vi "Assert Not Equal Value and Type_Variant.vi"(4 "Execution time (s)":dbl=-1.0, 6 "error code (1)":i32=1, 7 "Label":string, 8 "error in":errorcluster, 10 "Y":variant, 11 "X":variant) -> (0 "error out":errorcluster, 2 "Properties":refnum<class "Properties.Assert.lvclass">)   [LabVIEW 2021, in "Banana.Caraya.lvlib" / "Platano.CarayaTestSuite.lvclass"]
uses:
  Platano.CarayaTestSuite.lvclass
  Platano.CarayaTestSuite.lvclass/Platano.CarayaTestSuite.ctl
  <vilib>/addons/_JKI Toolkits/Caraya/classes/Assert/Assert.lvclass
  Bananas/Platano/Platano.lvclass
  Bananas/Banana/Banana.lvclass
  Bananas/AssertEqualType/AssertEqualType.lvclass
  Bananas/AssertEqualValue/AssertEqualValue.lvclass
  Properties.Banana/Properties.Banana.lvclass
  <vilib>/addons/_JKI Toolkits/Caraya/classes/Properties.Assert/Properties.Assert.lvclass
  C:/Program Files (x86)/National Instruments/LabVIEW 2021/vi.lib/addons/_JKI Toolkits/Caraya/classes/Properties/Properties.lvclass
  C:/Program Files (x86)/National Instruments/LabVIEW 2021/vi.lib/addons/_JKI Toolkits/Caraya/classes/Properties.Assert/Properties.Assert.lvclass
  C:/Repositories/LVOS/Bananas/lv-src/Bananas/AssertEqualValue/AssertEqualValue.lvclass
  C:/Repositories/LVOS/Bananas/lv-src/Bananas/BananaPeel/BananaPeel.lvclass
  C:/Repositories/LVOS/Bananas/lv-src/Bananas/AssertEqualType/AssertEqualType.lvclass
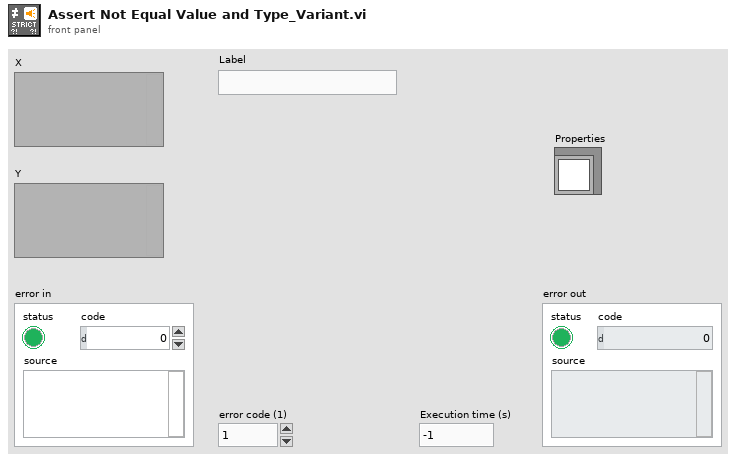
[diagram p1: front panel]
types:
  T1 = typedef "Bananas.lvlib/Assertion Strategies -- cluster.ctl" = cluster{"AssertTrue":refnum<class "AssertTrue.lvclass">, "AssertFalse":refnum<class "AssertFalse.lvclass">, "AssertEqualValue":refnum<class "AssertEqualValue.lvclass">, "AssertEqualType":refnum<class "AssertEqualType.lvclass">, "AssertCompareValue":refnum<class "AssertCompareValue.lvclass">, "AssertError":refnum<class "AssertError.lvclass">, "AssertAlmostEqual":refnum<class "AssertAlmostEqualValue.lvclass">}
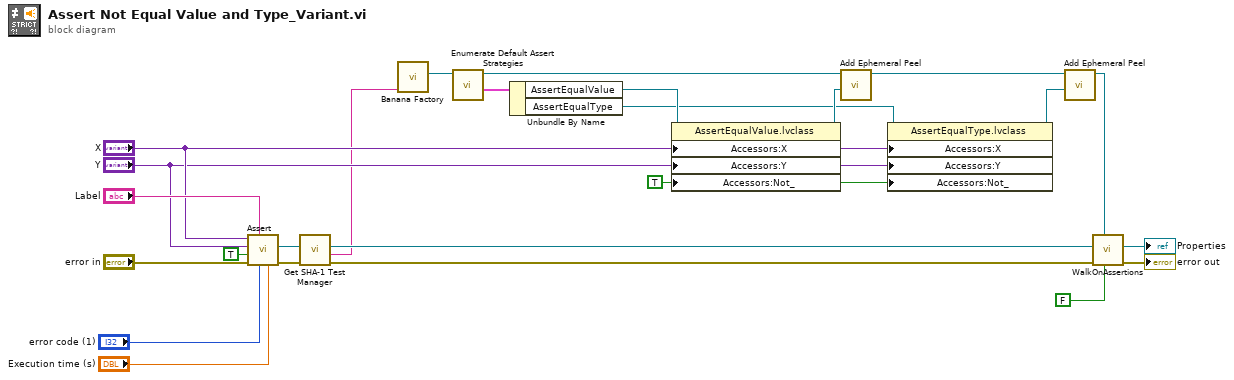
[diagram p0: block diagram]
diagram:
  w11 = TRUE ("Not_")
  n1 = call-poly <vilib>:"Assert.vi"("Execution time (s)"="Execution time (s)", "error code (1)"="error code (1)", "Label"="Label", "error in (no error)"="error in", "Register with caller test (F)"=TRUE, "Y"="Y", "X"="X") -> ("error out"=w6:errorcluster, "Properties.Assert"=w4:refnum<class "Properties.Assert.lvclass">)  [unwired: 3 in]
  n2 = call "Get SHA-1 Test Manager.vi"("error in (no error)"=w6, "Properties"=w4) -> ("error out"=w5:errorcluster, "SHA-1 hash"=w2:string, "Properties"=w3:refnum<class "Properties.Assert.lvclass">)  [unwired: 7 in]
  n3 = call "Banana Factory.vi"("Varietal"=w2) -> ("Banana"=w1:refnum<class "Banana.lvclass">)  [unwired: 9 in, 1 out]
  n4 = call "Enumerate Default Assert Strategies.vi"("Banana"=w1) -> ("Strategies"=w17:T1, "Banana"=w18:refnum<class "Banana.lvclass">)  [unwired: 9 in]
  n5 = Unbundle By Name(w17) -> ("AssertEqualValue"=w15:refnum<class "AssertEqualValue.lvclass">, "AssertEqualType"=w13:refnum<class "AssertEqualType.lvclass">)
  n6 = property class="AssertEqualValue.lvclass"(reference=w15, "Accessors:X"="X", "Accessors:Y"="Y", "Accessors:Not_"=w11) -> (reference out=w14:refnum<class "AssertEqualValue.lvclass">)  [unwired: 1 in, 1 out]
  n7 = call "Add Ephemeral Peel.vi"("BananaPeel"=w14, "Banana"=w18) -> ("Banana"=w16:refnum<class "Banana.lvclass">)  [unwired: 9 in]
  n8 = property class="AssertEqualType.lvclass"(reference=w13, "Accessors:X"="X", "Accessors:Y"="Y", "Accessors:Not_"=w11) -> (reference out=w12:refnum<class "AssertEqualType.lvclass">)  [unwired: 1 in, 1 out]
  n9 = call "Add Ephemeral Peel.vi"("BananaPeel"=w12, "Banana"=w16) -> ("Banana"=w8:refnum<class "Banana.lvclass">)  [unwired: 9 in]
  n10 = call "WalkOnAssertions.vi"("Stop on 1st fail"=FALSE, "Banana"=w8, "error in (no error)"=w5, "Properties"=w3) -> ("error out"=→"error out":errorcluster, "Properties out"=→"Properties":refnum<class "Properties.Assert.lvclass">)  [unwired: 6 in]
